vi "5_字符识别.vi"() -> ()   [LabVIEW 2020]
uses:
  <vilib>/vision/driver/NI_Vision_Acquisition_Software.lvlib
  <vilib>/vision/NI_Vision_Development_Module.lvlib
panel:
  out "Image":T1(plugin-control)
  out "Read String":string
  in  "Rectangle":T2 {"Rotation" min=-90.0 max=90.0 step=1.0 format="%.2f"; "Left" scale=0.0..1024.0; "Right" scale=0.0..1024.0}
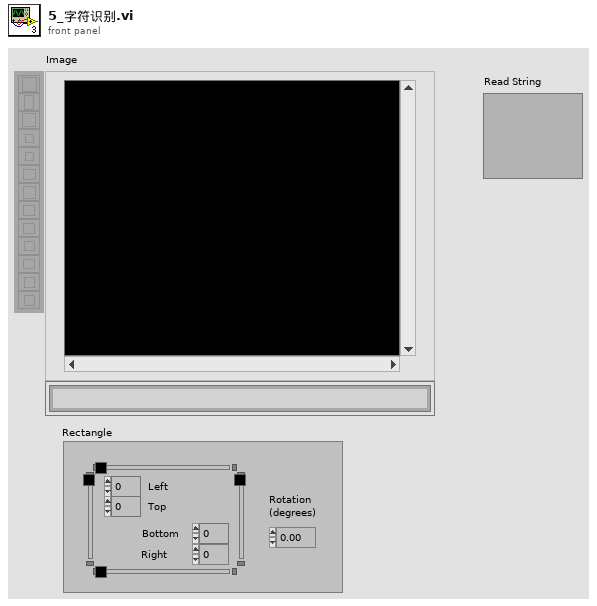
[diagram p1: front panel]
types:
  T1 = typedef "IMAQ Image.ctl" = refnum<image>
  T2 = typedef "IMAQ Rectangle" = cluster{"Left":i32, "Top":i32, "Right":i32, "Bottom":i32, "Rotation":dbl}
  T3 = typedef "IMAQ OCR Session.ctl" = refnum<k1>
  T4 = typedef "ROI Descriptor" = cluster{"Global Rectangle":i32[], "Contours":cluster{"ID":enum32{"External", "Internal"}, "Type":u32, "Coordinates":i32[]}[]}
  T5 = cluster{"Global Rectangle":i32[], "Contours":cluster{"ID":enum32{"External", "Internal"}, "Type":u32, "Coordinates":i32[]}[]}
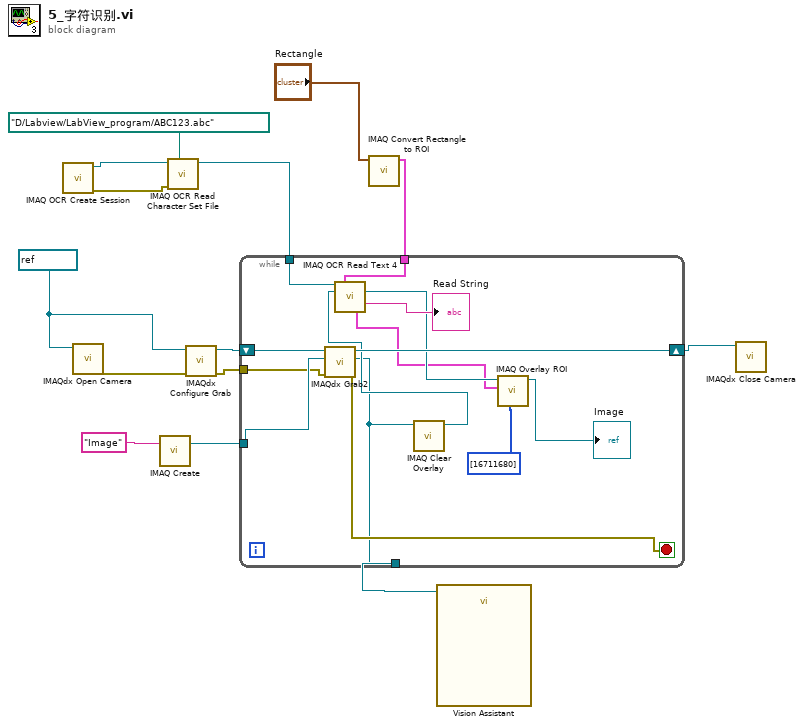
[diagram p0: block diagram]
diagram:
  w10 = refnum<k21> "cam1" ("Session In")
  n1 = call "IMAQ OCR Create Session"() -> ("error out"=w8:errorcluster, "IMAQ OCR Session"=w9:T3)  [unwired: 10 in]
  n2 = call <vilib>:"IMAQdx Open Camera.vi"("Session In"=w10) -> ("error out"=w14:errorcluster)  [unwired: 9 in, 1 out]
  n3 = call "IMAQ Create"("Image Name"="Image") -> ("New Image"=w4:T1)  [unwired: 4 in, 1 out]
  n4 = call "IMAQ OCR Read Character Set File"("File Path"=path "D:/Labview/LabView_program/ABC123.abc", "error in (no error)"=w8, "IMAQ OCR Session"=w9) -> ("IMAQ OCR Session (dup)"=w6:T3)  [unwired: 6 in, 2 out]
  n5 = call <vilib>:"IMAQdx Configure Grab.vi"("error in"=w14, "Session In"=w10) -> ("error out"=w1:errorcluster, "Session Out"=w13:refnum<k21>)  [unwired: 8 in]
  n6 = call "IMAQ Convert Rectangle to ROI"("Rectangle"="Rectangle") -> ("ROI Descriptor"=w2:T4)  [unwired: 8 in, 1 out]
  n7 = while {
    tunnel: w4 -> [w26]
    shift-right: [w27] -> w12
    shift-left: w13 -> [w28]
    tunnel: w6 -> [w25]
    tunnel: [w18] -> w3
    tunnel: w2 -> [w16]
    tunnel: w1 -> [w15]
    stop <- w23 stop-if-true
    n8 = call <vilib>:"IMAQdx Grab2.vi"("error in"=w15, "Image In"=w26, "Session In"=w28) -> ("error out"=w23:errorcluster, "Image Out"=w18:T1, "Session Out"=w27:refnum<k21>)  [unwired: 5 in, 1 out]
    n9 = call "IMAQ Clear Overlay"("Image"=w18) -> ("Image Out"=w19:T1)  [unwired: 9 in, 1 out]
    n10 = call "IMAQ OCR Read Text 4"("IMAQ OCR Session"=w25, "ROI Descriptor"=w16, "Image"=w19) -> ("Image (dup)"=w22:T1, "Read String"=→"Read String":string, "ROI Bounding Characters"=w20:T5)  [unwired: 6 in, 4 out]
    n11 = call "IMAQ Overlay ROI"("Colors (Green)"=u32[] [16711680], "ROI Descriptor"=w20, "Image"=w22) -> ("Image Out"=→"Image":T1)  [unwired: 7 in, 1 out]
  }
  n12 = call "Vision Assistant"("Image In"=w3) -> ()  [unwired: 25 in, 2 out]
  n13 = call <vilib>:"IMAQdx Close Camera.vi"("Session In"=w12) -> ()  [unwired: 10 in, 1 out]
